vi "TimeStamped CSV File Creation v2.0.vi"(8 "error in":errorcluster, 10 "Name Convention":string, 11 "Base Directory":path) -> (0 "error out":errorcluster, 3 "path":path)   [LabVIEW 2017]
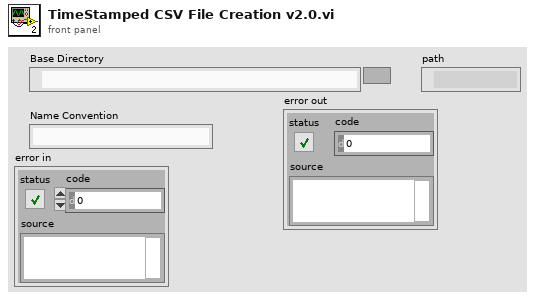
[diagram p1: front panel]
types:
  T1 = enum16{"open", "replace", "create", "open or create", "replace or create", "replace or create with confirmation"}
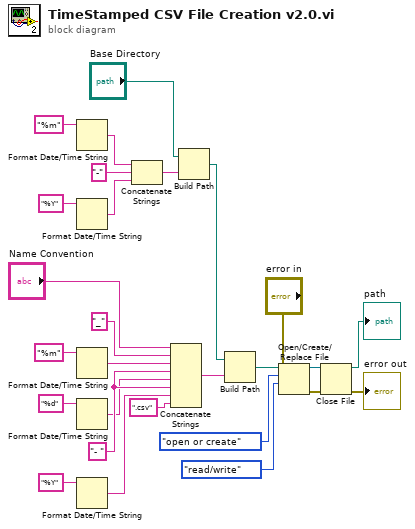
[diagram p0: block diagram]
diagram:
  w26 = "- " ("string")
  n1 = Format Date/Time String(time format string (%c)="%m") -> (date/time string=w7:string)  [unwired: 2 in]
  n2 = Format Date/Time String(time format string (%c)="%Y") -> (date/time string=w5:string)  [unwired: 2 in]
  n3 = Format Date/Time String(time format string (%c)="%m") -> (date/time string=w21:string)  [unwired: 2 in]
  n4 = Format Date/Time String(time format string (%c)="%d") -> (date/time string=w14:string)  [unwired: 2 in]
  n5 = Format Date/Time String(time format string (%c)="%Y") -> (date/time string=w15:string)  [unwired: 2 in]
  n6 = Concatenate Strings(w7, "-" ("string"), w5) -> (w4:string)
  n7 = Concatenate Strings("Name Convention", "_" ("string"), w21, w26, w14, w26, w15, ".csv" ("string")) -> (w23:string)
  n8 = Build Path(base path="Base Directory", name or relative path=w4) -> (appended path=w2:path)
  n9 = Build Path(base path=w2, name or relative path=w23) -> (appended path=w16:path)
  n10 = Open/Create/Replace File(file path (use dialog)=w16, error in="error in", operation (0:open)=T1."open or create", access (0:read/write)=enum16{"read/write", "read-only", "write-only"}."read/write") -> (refnum out=w20:refnum<file>, error out=w19:errorcluster)  [unwired: 2 in, 1 out]
  n11 = Close File(refnum=w20, error in=w19) -> (path=→"path":path, error out=→"error out":errorcluster)
